vi "get errno pointer for calling thread.vi"(8 "error in (no error)":errorcluster) -> (0 "error out":errorcluster, 3 "errno pointer":u64 format="0x%016x")   [LabVIEW 2013, in "Linux Errno.lvlib"]
uses:
  Linux Errno.lvlib
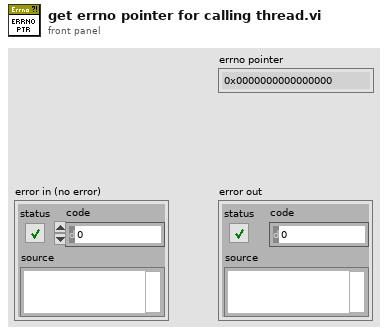
[diagram p1: front panel]
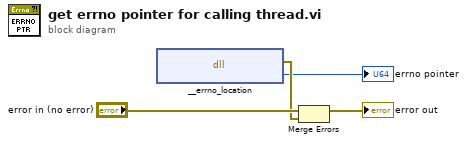
[diagram p0: block diagram]
diagram:
  n1 = dll-call lib="LabVIEW" fn="__errno_location"() -> (error out=w3:errorcluster, "return type"=→"errno pointer":u64)  [unwired: 3 in, 1 out]
  n2 = Merge Errors("error in (no error)", w3) -> (→"error out":errorcluster)
